vi "Write String.vi"(6 "error in (no error)":errorcluster, 7 "Bus In":refnum<class "Bus.lvclass">, 8 "Channel Name":string, 9 "Data Value Engineering":dbl, 10 "Data Value Native":dbl, 11 "NI Digital in":refnum<class "Single Channel.lvclass">) -> (0 "error out":errorcluster, 3 "NI Digital out":refnum<class "Single Channel.lvclass">, 5 "Bus Out":refnum<class "Bus.lvclass">)   [LabVIEW 2018, in "Single Channel.lvclass"]
doc: "String Out.lvclass:Read String.vi\n\nThis is the template for the Read String VI forthe String Out class.\n\nInstrument Communication Module Version 1.0\nOctober, 2020 Original Code Consulting Davita Bird\n www.originalcode.com"
uses:
  Single Channel.lvclass
  Bus/Bus.lvclass
  Single Channel.lvclass/Single Channel.ctl
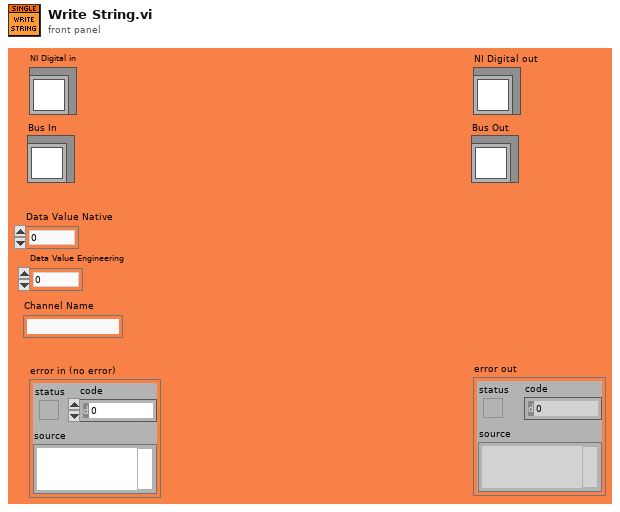
[diagram p1: front panel]
types:
  T1 = cluster{"Parsing String":string, "Channel Name":string, "Enabled":bool, "Initial Value":dbl}[]
  T2 = cluster{"Parsing String":string, "Channel Name":string, "Enabled":bool, "Initial Value":dbl}
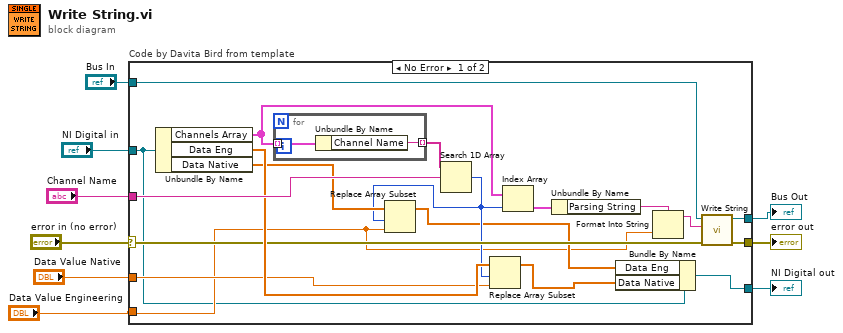
[diagram p0: block diagram]
diagram:
  n1 = case "Code by Davita Bird from template" shown="No Error" "error in (no error)" {
    selector: "error in (no error)" -> [w17 w33]
    tunnel: [w26 w33] -> w8
    tunnel: [w16 w32] -> w7
    tunnel: "NI Digital in" -> [w10 w32]
    tunnel: "Data Value Native" -> [w23 _]
    tunnel: "Bus In" -> [w27 w31]
    tunnel: [w28 w31] -> w4
    tunnel: "Channel Name" -> [w25 _]
    tunnel: "Data Value Engineering" -> [w12 _]
    frame No Error {
      n2 = Unbundle By Name(w10) -> ("Channels Array"=w20:T1, "Data Eng"=w24:dbl[], "Data Native"=w15:dbl[])
      n3 = for {
        tunnel: w20 -> [w30] mode=indexing
        tunnel: [w29] -> w21 mode=indexing
        n4 = Unbundle By Name(w30) -> ("Channel Name"=w29:string)
      }
      n5 = Search 1D Array(1D array=w21, element=w25) -> (index of element=w14:i32)  [unwired: 1 in]
      n6 = Replace Array Subset(array=w15, new element=w12, index=w14) -> (w13:dbl[])
      n7 = Replace Array Subset(array=w24, new element=w23, index=w14) -> (w11:dbl[])
      n8 = Index Array(array=w20, index=w14) -> (element=w18:T2)
      n9 = Unbundle By Name(w18) -> ("Parsing String"=w19:string)
      n10 = Bundle By Name(cluster=w10, "Data Eng"=w13, "Data Native"=w11) -> (w16:refnum<class "Single Channel.lvclass">)
      n11 = Format Into String(format string=w19, w12) -> (resulting string=w22:string)  [unwired: 2 in, 1 out]
      n12 = call-dynamic "Write String.vi"("error in (no error)"=w17, "String"=w22, "Bus in"=w27) -> ("error out"=w26:errorcluster, "Bus out"=w28:refnum<class "Bus.lvclass">)  [unwired: 7 in]
    }
    frame Error {
    }
  }
  "error out" <- w8
  "NI Digital out" <- w7
  "Bus Out" <- w4
